vi "Configure Motor.vi"   [LabVIEW 2021, in "Yokogawa WT1800 Series.lvlib"]
doc: "Configures the motor features.\n\n<b>Note:</b>\nThis setting valid on models with the motor evaluation function (/MTR) option."
uses:
  <instrlib>/Yokogawa WT1800 Series/Yokogawa WT1800 Series.lvlib
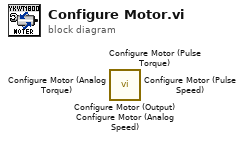
[diagram p0: block diagram]
diagram:
  n1 = call <instrlib>:"Configure Motor (Output).vi"() -> ()  [unwired: 14 in, 2 out]
  n2 = call <instrlib>:"Configure Motor (Pulse Torque).vi"() -> ()  [unwired: 14 in, 2 out]
  n3 = call <instrlib>:"Configure Motor (Analog Torque).vi"() -> ()  [unwired: 14 in, 2 out]
  n4 = call <instrlib>:"Configure Motor (Pulse Speed).vi"() -> ()  [unwired: 14 in, 2 out]
  n5 = call <instrlib>:"Configure Motor (Analog Speed).vi"() -> ()  [unwired: 14 in, 2 out]
